vi "Configure AC Voltage Range Mode.vi"(0 "VISA resource name":refnum<visa-resource-name>, 5 "Voltage Range Mode (1:Auto)":u16(ring)=1 items=["High", "Auto"], 11 "error in (no error)":errorcluster) -> (4 "VISA resource name out":refnum<visa-resource-name>, 15 "error out":errorcluster)   [LabVIEW 2020, in "eec 6700.lvlib"]
doc: "Sets the <B>Range Mode</B> of the AC voltage</B> in the active step of the power source instrument.\n\n<B>For AC</B>: High | Auto\n\nVoltage Mode indicates whether the instrument is in the AUTO or HIGH mode.\nSetting the Voltage Mode to AUTO, the system will automatically interpret the voltage range and switch to the high or low voltage output range.\nSetting the Voltage Mode to HIGH will put the output voltage into the high voltage output range and the current is limited to half as compared to the current limit in the low voltage output range.\n(Refer to the specification table regarding current output based on voltage output range).\nSetting of voltage range may not influence the existing output voltage setting."
uses:
  <instrlib>/EEC6700LV-driver/eec 6700.lvlib
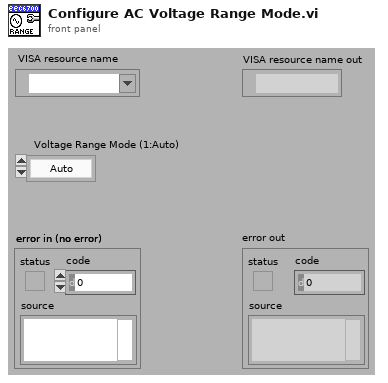
[diagram p1: front panel]
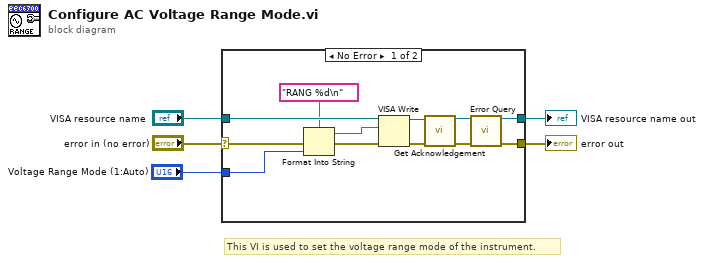
[diagram p0: block diagram]
diagram:
  # "This VI is used to set the voltage range mode of the instrument."
  n1 = case shown="No Error" "error in (no error)" {
    selector: "error in (no error)" -> [w12 w19]
    tunnel: "VISA resource name" -> [w17 w18]
    tunnel: [w14 w18] -> w4
    tunnel: [w13 w19] -> w3
    tunnel: "Voltage Range Mode (1:Auto)" -> [w10 _]
    frame No Error {
      n2 = Format Into String(format string="RANG %d\n" ("Command"), error in=w12, w10) -> (resulting string=w15:string, error out=w11:errorcluster)  [unwired: 1 in]
      n3 = VISA Write(VISA resource name=w17, write buffer=w15, error in (no error)=w11) -> (VISA resource name out=w7:refnum<visa-resource-name>, error out=w8:errorcluster)  [unwired: 1 out]
      n4 = call <instrlib>:"Get Acknowledgement.vi"("VISA resource name"=w7, "error in (no error)"=w8) -> ("VISA resource name out"=w6:refnum<visa-resource-name>, "error out"=w9:errorcluster)  [unwired: 12 in]
      n5 = call <instrlib>:"Error Query.vi"("VISA resource name"=w6, "error in (no error)"=w9) -> ("VISA resource name out"=w14:refnum<visa-resource-name>, "error out"=w13:errorcluster)  [unwired: 10 in, 2 out]
    }
    frame Error {
    }
  }
  "error out" <- w3
  "VISA resource name out" <- w4
